vi "Main.vi"(10 "JQMHStartup.lvclass":refnum<class "RQMHStartup.lvclass">, 11 "JQMHCore in":refnum<class "RQMHModule.lvclass">) -> ()   [LabVIEW 2024, in "RQMHModule.lvclass"]
uses:
  RQMHModule.lvclass
  Startup/RQMHStartup.lvclass
  Startup/Command.ctl
  RQMHModule.lvclass/RQMHModule.ctl
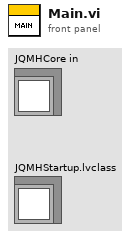
[diagram p1: front panel]
types:
  T1 = typedef "RQMHStartup.lvclass/Command.ctl" = enum16{"Default", "No Override", "Error", "ACK Created", "ACK Mod Reg", "ACK Caller Reg"}
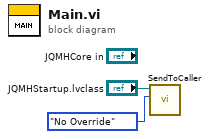
[diagram p0: block diagram]
diagram:
  n1 = call "SendToCaller.vi"("Command"=Command."No Override", "JQMHStartup in"="JQMHStartup.lvclass") -> ()  [unwired: 8 in, 2 out]
